vi "ListoEvaluar.vi"(8 "error in (no error)":errorcluster, 11 "Prueba21 in":refnum<class "Prueba21.lvclass">) -> (0 "error out":errorcluster, 2 "listo_para_evaluar":bool, 3 "Prueba21 out":refnum<class "Prueba21.lvclass">)   [LabVIEW 2019, in "Prueba21.lvclass"]
uses:
  Prueba21.lvclass
  Prueba21.lvclass/Prueba21.ctl
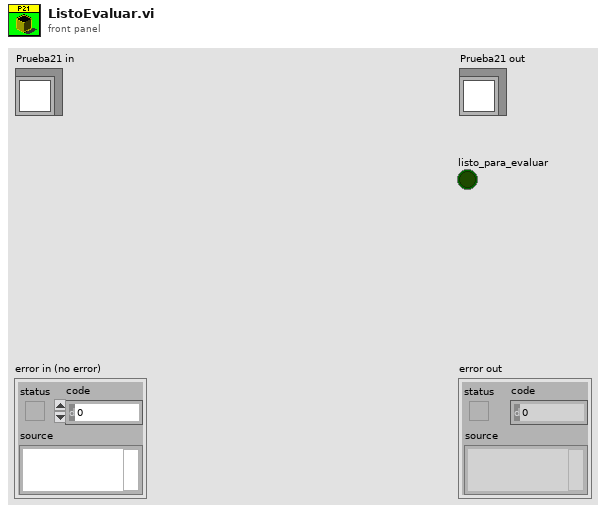
[diagram p1: front panel]
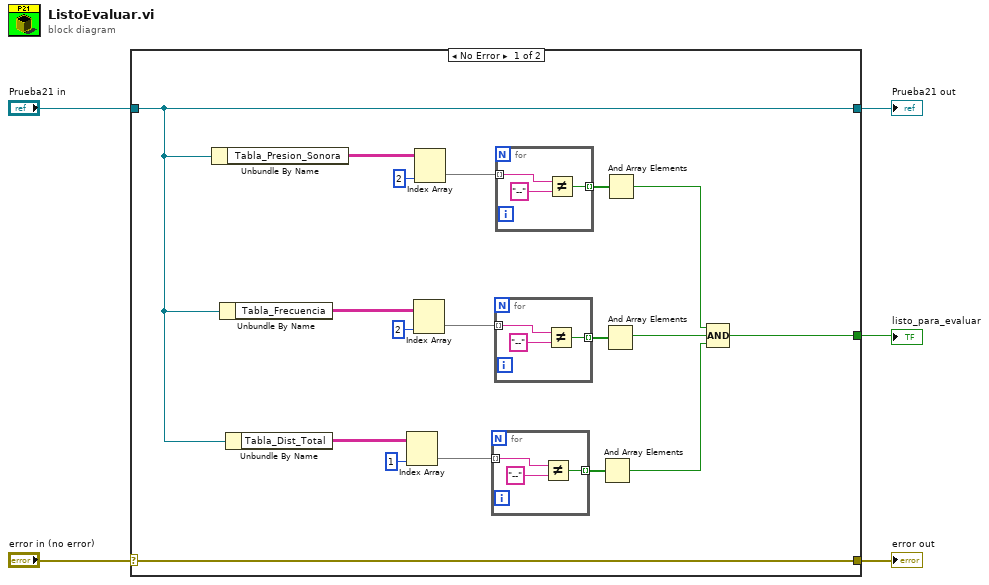
[diagram p0: block diagram]
diagram:
  n1 = case shown="No Error" "error in (no error)" {
    selector: "error in (no error)" -> [w23 w34]
    tunnel: [w23 w34] -> w4
    tunnel: [w22 w33] -> w2
    tunnel: "Prueba21 in" -> [w22 w33]
    tunnel: [w6 _] -> w1
    frame No Error {
      n2 = Unbundle By Name(w22) -> ("Tabla_Presion_Sonora"=w21:string[][])
      n3 = Unbundle By Name(w22) -> ("Tabla_Frecuencia"=w17:string[][])
      n4 = Unbundle By Name(w22) -> ("Tabla_Dist_Total"=w16:string[][])
      n5 = Index Array(array=w16, index (col)=1 ("disabled index (col)")) -> (element=w10:string[])  [unwired: 1 in]
      n6 = Index Array(array=w17, index (col)=2 ("disabled index (col)")) -> (element=w11:string[])  [unwired: 1 in]
      n7 = Index Array(array=w21, index (col)=2 ("disabled index (col)")) -> (element=w14:string[])  [unwired: 1 in]
      n8 = for {
        tunnel: [w26] -> w12 mode=indexing
        tunnel: w10 -> [w24] mode=indexing
        n9 = Not Equal?(x=w24, y="--") -> (x != y?=w26:bool)
      }
      n10 = for {
        tunnel: [w29] -> w13 mode=indexing
        tunnel: w11 -> [w27] mode=indexing
        n11 = Not Equal?(x=w27, y="--") -> (x != y?=w29:bool)
      }
      n12 = for {
        tunnel: [w32] -> w15 mode=indexing
        tunnel: w14 -> [w30] mode=indexing
        n13 = Not Equal?(x=w30, y="--") -> (x != y?=w32:bool)
      }
      n14 = And Array Elements(Boolean array=w12) -> (logical AND=w7:bool)
      n15 = And Array Elements(Boolean array=w13) -> (logical AND=w8:bool)
      n16 = And Array Elements(Boolean array=w15) -> (logical AND=w9:bool)
      n17 = Compound Arithmetic op=AND(w9, w8, w7) -> (w6:bool)
    }
    frame Error {
    }
  }
  "error out" <- w4
  "Prueba21 out" <- w2
  "listo_para_evaluar" <- w1
